vi "D_A Output Source.vi"(7 "Read Value? (F)":bool, 8 "error in (no error)":errorcluster, 10 "Output Source (A)":T1, 11 "VISA resource name":refnum<visa-resource-name>) -> (0 "error out":errorcluster, 2 "Output Source":T1, 3 "VISA resource name out":refnum<visa-resource-name>)   [LabVIEW 2013, in "SRS SR400.lvlib"]
doc: "<B>AS { j }</B>\n\nThe AS command reads and sets the front panel D/A output source. If j is absent, the D/A source is returned. The parameter j may only be included if the counting mode is A,B FOR T PRESET. In this case, j=0 or 1 selects A or B. In all other modes, the D/A output follows the count display. The source may be read in all modes.\n\n<B>j</B> <B>Output source</B>\n0 A\n1 B\n2 A-B\n3 A+B"
uses:
  <instrlib>/SRS SR400/SRS SR400.lvlib
  <instrlib>/SRS SR400/Public/Typedefs/Output Source.ctl
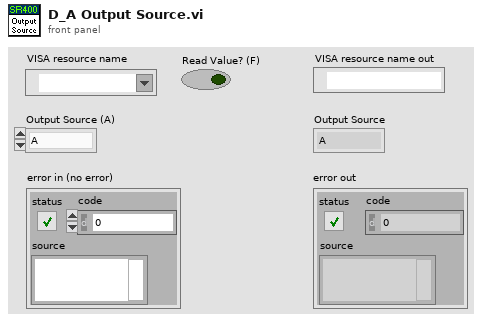
[diagram p1: front panel]
types:
  T1 = typedef "SRS SR400.lvlib/Output Source.ctl" = enum16{"A", "B", "A - B", "A + B"}
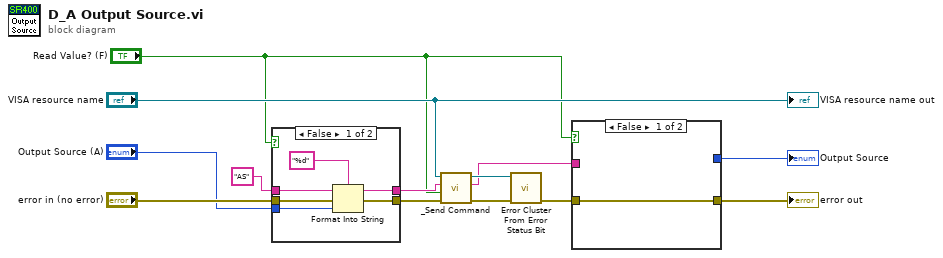
[diagram p0: block diagram]
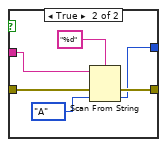
[diagram p2: hidden frame]
diagram:
  n1 = case shown="False" "Read Value? (F)" {
    tunnel: "error in (no error)" -> [w19 w21]
    tunnel: "AS" ("command") -> [w17 w20]
    tunnel: [w16 w20] -> w11
    tunnel: [w15 w21] -> w10
    tunnel: "Output Source (A)" -> [w14 _]
    frame False {
      n2 = Format Into String(format string="%d", initial string=w17, error in=w19, w14) -> (resulting string=w16:string, error out=w15:errorcluster)
    }
    frame True {
    }
  }
  n3 = call <instrlib>:"_Send Command.vi"("error in (no error)"=w10, "Read Value? (F)"="Read Value? (F)", "Command"=w11, "VISA resource name"="VISA resource name") -> ("error out"=w7:errorcluster, "Response"=w4:string, "VISA resource name out"=w8:refnum<visa-resource-name>)  [unwired: 5 out]
  n4 = call <instrlib>:"Error Cluster From Error Status Bit.vi"("error in (no error)"=w7, "VISA resource name"=w8) -> ("error out"=w5:errorcluster)  [unwired: 8 in, 1 out]
  n5 = case shown="False" "Read Value? (F)" {
    tunnel: w5 -> [w22 w28]
    tunnel: w4 -> [_ w26]
    tunnel: [w22 w24] -> w2
    tunnel: [_ w23] -> w1
    frame False {
    }
    frame True {
      n6 = Scan From String(format string="%d", input string=w26, error in=w28, default 1=Output_Source."A" ("Output Source (A)")) -> (error out=w24:errorcluster, output 1=w23:T1)  [unwired: 1 in, 2 out]
    }
  }
  "error out" <- w2
  "Output Source" <- w1
  "VISA resource name out" <- "VISA resource name"
